vi "Create interprocess data queues.vi"(8 "error in (no error)":errorcluster, 11 "Application in":refnum<class "Application.lvclass">) -> (0 "error out":errorcluster, 1 "RawDaqDataQ":T1, 2 "InverterWaveformsQ":T2, 3 "Application out":refnum<class "Application.lvclass">)   [LabVIEW 2019, in "Application.lvclass"]
doc: "Developed by Kevin Thompson\nkevin@thompsonengineering.net\n\nCopyright 2020\nThompson Engineering, LLC"
uses:
  Application.lvclass
  Common/DataTypes/ChannelWaveforms--cluster.ctl
  Common/DataTypes/InverterWaveforms--cluster.ctl
  Common/DataTypes/InverterWaveforms--QRef.ctl
  Common/DataTypes/RawChannelData--cluster.ctl
  Common/DataTypes/RawDAQData--cluster.ctl
  Common/DataTypes/RawDAQDataQRef--cluster.ctl
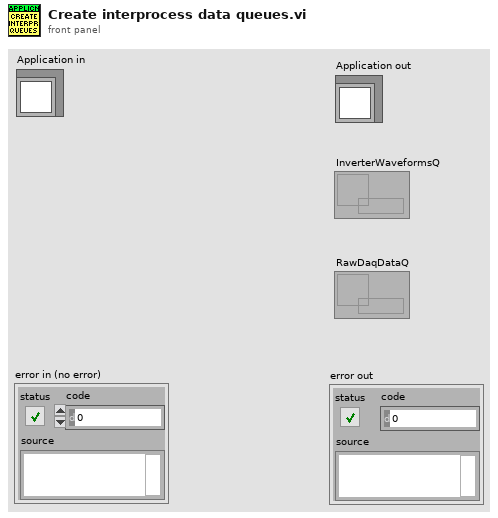
[diagram p1: front panel]
types:
  T1 = typedef "RawDAQDataQRef--cluster.ctl" = refnum<queue>
  T2 = typedef "InverterWaveforms--QRef.ctl" = refnum<queue>
  T3 = typedef "RawDAQData--cluster.ctl" = cluster{"Module1-2_9775":T4, "Module 3-4_9215":T4}
  T4 = typedef "RawChannelData--cluster.ctl" = cluster{"TS":timestamp, "ScanArray":dbl[]}
  T5 = typedef "InverterWaveforms--cluster.ctl" = T6[]
  T6 = typedef "ChannelWaveforms--cluster.ctl" = cluster{"Iin ripple ":waveform(dbl), "Iout ripple ":waveform(dbl), "Vout 60Hz":waveform(dbl), "Iout 60Hz":waveform(dbl)}
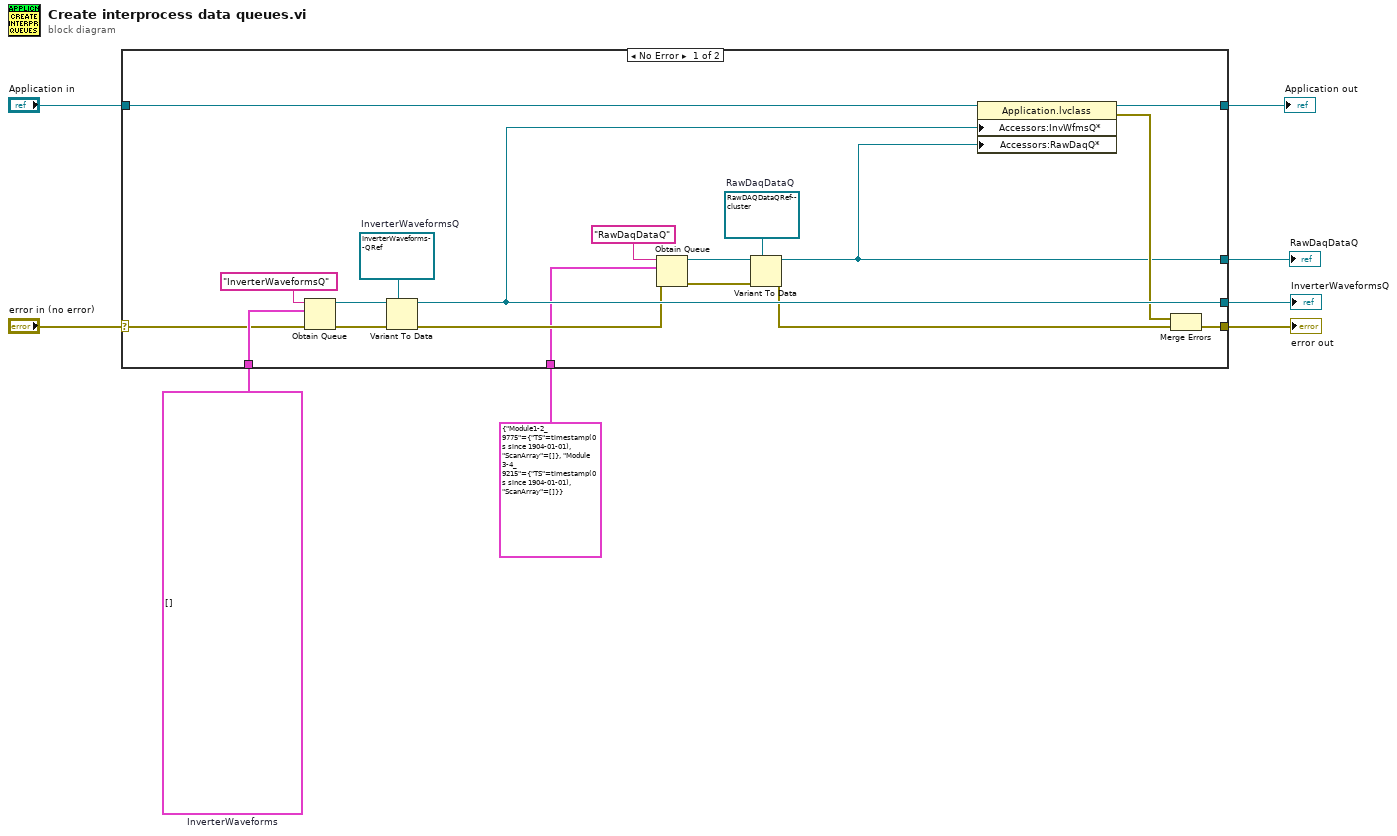
[diagram p0: block diagram]
diagram:
  w7 = T5 []  # InverterWaveforms
  n1 = case shown="No Error" "error in (no error)" {
    selector: "error in (no error)" -> [w23 w29]
    tunnel: [w20 _] -> w8
    tunnel: w7 -> [w26 _]
    tunnel: [w19 w29] -> w6
    tunnel: "Application in" -> [w22 w28]
    tunnel: [w21 w28] -> w3
    tunnel: T3 {"Module1-2_9775"={"TS"=timestamp(0 s since 1904-01-01), "ScanArray"=[]}, "Module 3-4_9215"={"TS"=timestamp(0 s since 1904-01-01), "ScanArray"=[]}} ("RawDAQData") -> [w14 _]
    tunnel: [w11 _] -> w1
    frame No Error {
      w12 = T1 refnum  # RawDaqDataQ
      w25 = T2 refnum  # InverterWaveformsQ
      n2 = Obtain Queue(name (unnamed)="InverterWaveformsQ", element data type=w26, error in (no error)=w23) -> (queue out=w27:refnum<queue>, error out=w24:errorcluster)  [unwired: 2 in, 1 out]
      n3 = Variant To Data(error in=w24, type=w25, Variant=w27) -> (data=w20:T2, error out=w15:errorcluster)
      n4 = Obtain Queue(name (unnamed)="RawDaqDataQ", element data type=w14, error in (no error)=w15) -> (queue out=w13:refnum<queue>, error out=w9:errorcluster)  [unwired: 2 in, 1 out]
      n5 = Variant To Data(error in=w9, type=w12, Variant=w13) -> (data=w11:T1, error out=w10:errorcluster)
      n6 = property class="Application.lvclass"(reference=w22, "Accessors:InvWfmsQ*"=w20, "Accessors:RawDaqQ*"=w11) -> (reference out=w21:refnum<class "Application.lvclass">, error out=w18:errorcluster)  [unwired: 1 in]
      n7 = Merge Errors(w18, w10) -> (w19:errorcluster)
    }
    frame Error {
    }
  }
  "InverterWaveformsQ" <- w8
  "error out" <- w6
  "Application out" <- w3
  "RawDaqDataQ" <- w1
